vi "Set Data.vi"(10 "Persistent":T1={"Initial Path"=path "", "INI Path"=path "", "INI Section"="Last Used", "Select Option?"=TRUE, "Explorer Option?"=TRUE, "Recurse?"=TRUE, "Allow New?"=FALSE, "Filter"="*.*"}, 11 "Persistent Path Selector in":refnum<class "MGI Persistent Path Selector.lvclass">) -> (3 "Persistent Path Selector out":refnum<class "MGI Persistent Path Selector.lvclass">)   [LabVIEW 2016, in "MGI Persistent Path Selector.lvclass"]
doc: "Set protected data."
uses:
  <userlib>/_MGI/User Interface/Path Selector XControl/Class Hierarchy/Persistent Path Selector/MGI Persistent Path Selector.lvclass
  <userlib>/_MGI/User Interface/Path Selector XControl/Class Hierarchy/Persistent Path Selector/Persistent Data Cluster.ctl
  <userlib>/_MGI/User Interface/Path Selector XControl/Class Hierarchy/Persistent Path Selector/MGI Persistent Path Selector.lvclass/MGI Persistent Path Selector.ctl
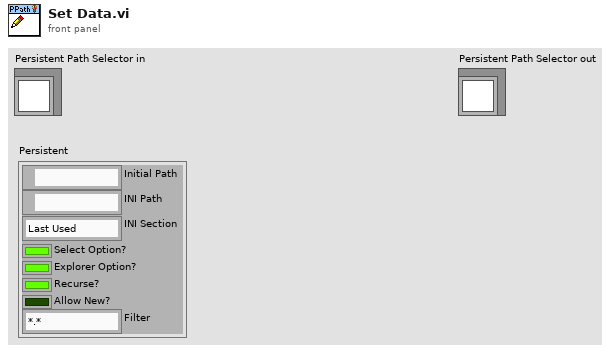
[diagram p1: front panel]
types:
  T1 = typedef "MGI Persistent Path Selector.lvclass/Persistent Data Cluster.ctl" = cluster{"Initial Path":path, "INI Path":path, "INI Section":string, "Select Option?":bool, "Explorer Option?":bool, "Recurse?":bool, "Allow New?":bool, "Filter":string}
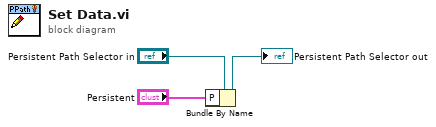
[diagram p0: block diagram]
diagram:
  n1 = Bundle By Name(cluster="Persistent Path Selector in", "P"="Persistent") -> (→"Persistent Path Selector out":refnum<class "MGI Persistent Path Selector.lvclass">)
